vi "Read data_create folder file.vi"(10 "name or relative path":string, 11 "path":path) -> (3 "dup path":path)   [LabVIEW 2016]
panel:
  out "error out":errorcluster
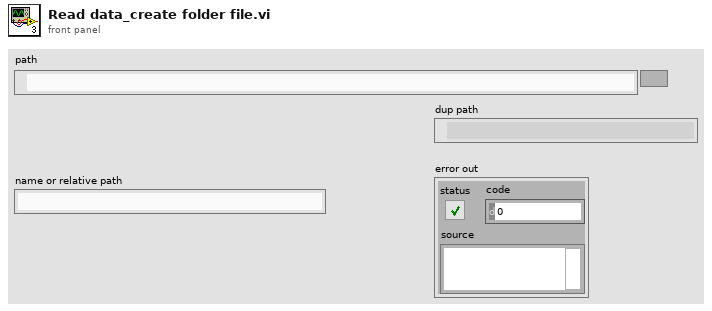
[diagram p1: front panel]
types:
  T1 = enum16{"open", "replace", "create", "open or create", "replace or create", "replace or create with confirmation"}
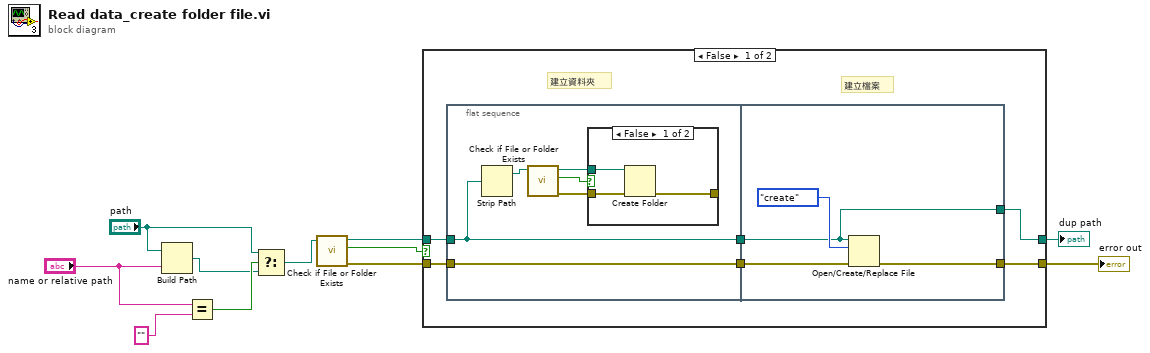
[diagram p0: block diagram]
diagram:
  n1 = Build Path(base path="path", name or relative path="name or relative path") -> (appended path=w2:path)
  n2 = Equal?(x="name or relative path", y="") -> (x = y?=w3:bool)
  n3 = Select(t="path", s=w3, f=w2) -> (s? t:f=w4:path)
  n4 = call <vilib>:"Check if File or Folder Exists.vi"("path"=w4) -> ("error out"=w9:errorcluster, "file or folder exists?"=w11:bool, "dup path"=w10:path)  [unwired: 8 in]
  n5 = case shown="False" w11 {
    tunnel: w10 -> [w16 w33]
    tunnel: w9 -> [w17 w32]
    tunnel: [w15 w32] -> w8
    tunnel: [w14 w33] -> w7
    frame False {
      # "建立檔案"
      # "建立資料夾"
      n6 = flat-sequence {
        tunnel: w16 -> [w18]
        tunnel: w17 -> [w23]
        tunnel: [w23] -> w13
        tunnel: [w18] -> w12
        tunnel: [w29] -> w15
        tunnel: [w28] -> w14
        tunnel: w13 -> [w30]
        tunnel: w12 -> [w28]
        frame #0 {
          n7 = Strip Path(path=w18) -> (stripped path=w19:path)  [unwired: 1 out]
          n8 = call <vilib>:"Check if File or Folder Exists.vi"("path"=w19) -> ("error out"=w22:errorcluster, "file or folder exists?"=w20:bool, "dup path"=w21:path)  [unwired: 8 in]
          n9 = case shown="False" w20 {
            tunnel: w21 -> [w26 _]
            tunnel: [w25 w27] -> _
            tunnel: w22 -> [w24 w27]
            frame False {
              n10 = Create Folder(path (use dialog)=w26, error in=w24) -> (error out=w25:errorcluster)  [unwired: 1 in, 2 out]
            }
            frame True {
            }
          }
        }
        frame #1 {
          n11 = Open/Create/Replace File(file path (use dialog)=w28, error in=w30, operation (0:open)=T1."create") -> (error out=w29:errorcluster)  [unwired: 3 in, 2 out]
        }
      }
    }
    frame True {
    }
  }
  "error out" <- w8
  "dup path" <- w7
